vi "convertReadResponse.vi"(8 "error in (no error)":errorcluster, 11 "rawDataIn":u8[](array[numeric])) -> (0 "error out":errorcluster, 1 "setValue":u16, 2 "cmd":u8, 3 "rawDataOut":u8[](array[numeric]))   [LabVIEW 2016]
doc: "Convert the LAC raw response to a distance\n\nFormat: 3-byte packet\nControl, Data Low, Data High\nBuffer[0]=Control\nBuffer[1]=Data Low\nBuffer[2]=Data High\n\nWritten by: Complete Automated Solutions\nwww.CompleteAutomatedSolutions.com"
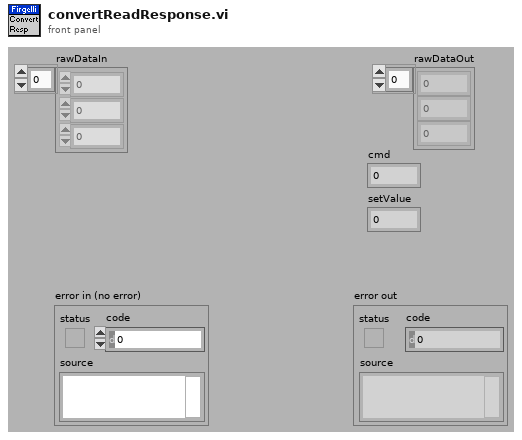
[diagram p1: front panel]
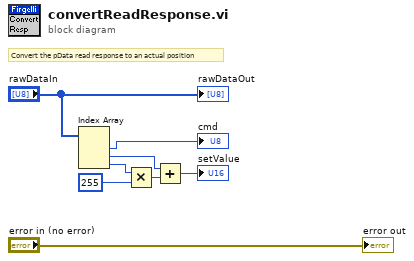
[diagram p0: block diagram]
diagram:
  # "Convert the pData read response to an actual position"
  n1 = Index Array(array="rawDataIn") -> (element #1=→"cmd":u8, element #2=w3:u8, element #3=w6:u8)  [unwired: 3 in]
  n2 = Multiply(x=w6, y=u16 255) -> (x*y=w4:u16)
  n3 = Add(x=w3, y=w4) -> (x+y=→"setValue":u16)
  "rawDataOut" <- "rawDataIn"
  "error out" <- "error in (no error)"
